vi "BotSpeak.Com.vi"(1 "To Send":string, 2 "Bot Settings in":T1) -> (3 "error out":errorcluster, 4 "Sent":string, 5 "Reply":string, 6 "Bot Settings out":T1)   [LabVIEW 2012]
uses:
  <userlib>/botspeak/VIs/Direct/BotSpeak_Control.ctl
  <userlib>/botspeak/VIs/SubVIs/BotSpeak_Globals.vi
panel:
  out "Numeric":i32
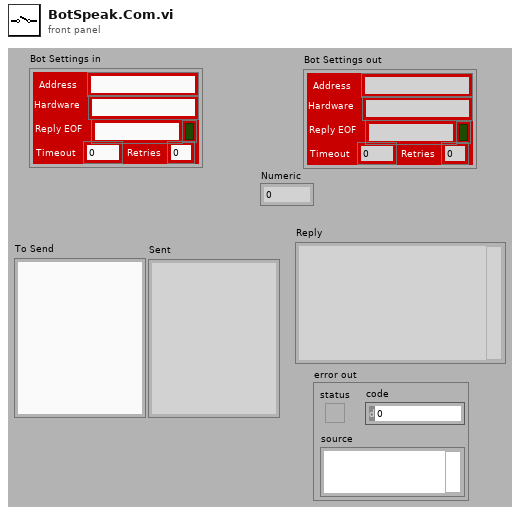
[diagram p1: front panel]
types:
  T1 = typedef "BotSpeak_Control.ctl" = cluster{"Address":string, "Reply EOF":string, "Hardware":string, "Retries":i8, "Timeout":i32, "Open?":bool}
  T2 = typedef "BotSpeak.HardwareSpecs.ctl" = cluster{"Hardware Name":string, "Hardware URL":string, "ComType":enum16{"Undefined", "HTTP", "Serial", "TCPIP", "Console"}, "TCP Port":i32, "DefaultAddress":string, "Retries":i32, "Translate":enum16{"None", "Tiny", "URAPI"}, "MaxScriptSize":i32, "MaxVarNumber":i32, "StartupWait":i32, "Patience":i32, "Startup Patience":i32, "Hardware Help":string, "Com Protocol":string, "Translator":cluster{"BotSpeak CMD":string, "CMD out":string}[], "Init Code":string, "Variable Format":enum16{"INT", "FLOAT", "FIXED"}, "username":string, "password":string}
  T3 = cluster{"BotSpeak CMD":string, "CMD out":string}[]
  T4 = enum16{"Undefined", "HTTP", "Serial", "TCPIP", "Console"}
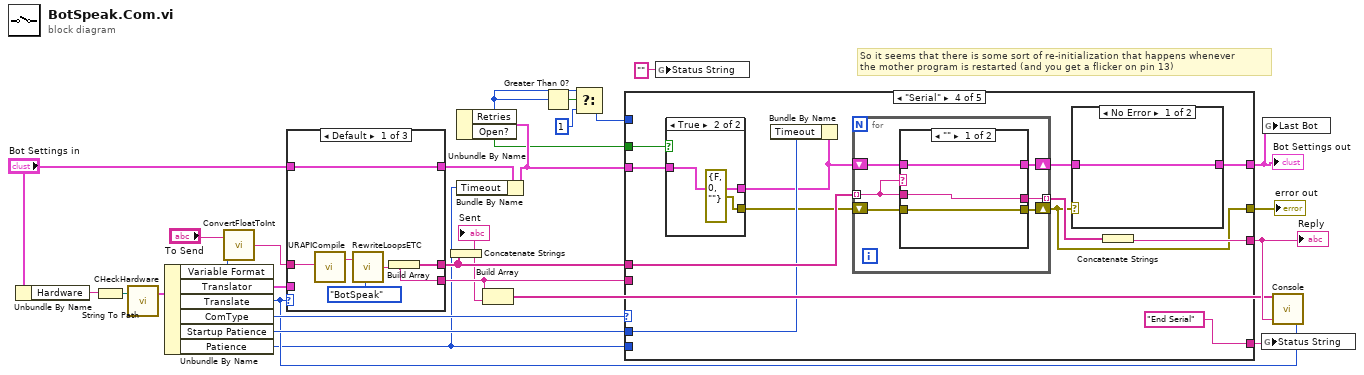
[diagram p0: block diagram]
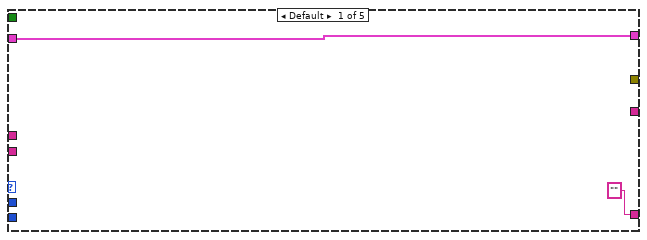
[diagram p2: hidden frame]
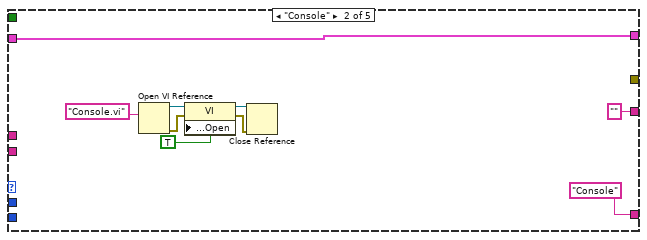
[diagram p3: hidden frame]
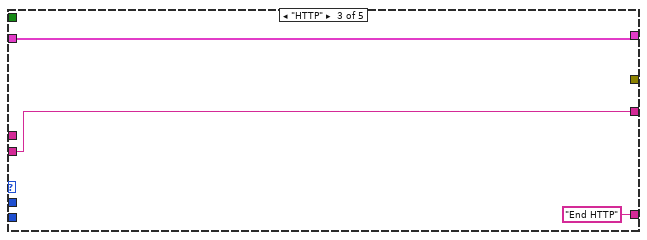
[diagram p4: hidden frame]
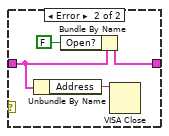
[diagram p5: hidden frame]
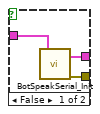
[diagram p6: hidden frame]
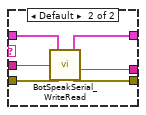
[diagram p7: hidden frame]
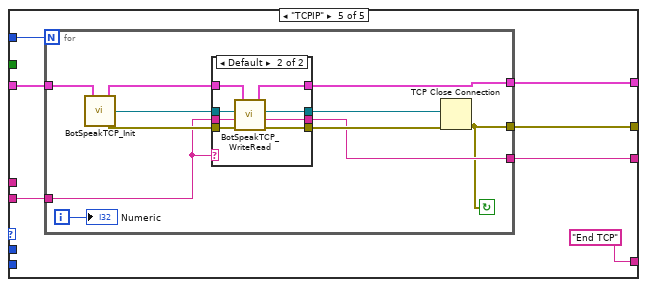
[diagram p8: hidden frame]
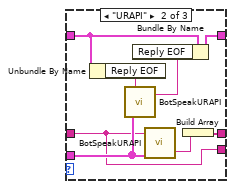
[diagram p10: hidden frame]
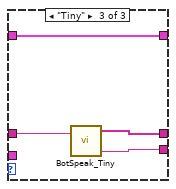
[diagram p11: hidden frame]
diagram:
  # "So it seems that there is some sort of re-initialization that happens whenever\nthe mother program is restarted (and you get a flicker on pin 13)"
  n1 = Unbundle By Name("Bot Settings in") -> ("Hardware"=w27:string)
  n2 = String To Path(string=w27) -> (path=w10:path)
  n3 = call <userlib>:"CHeckHardware.vi"("Hardware"=w10) -> ("HardwareSpecs"=w23:T2)  [unwired: 2 in]
  n4 = Unbundle By Name(w23) -> ("Variable Format"=w11:enum16{"INT", "FLOAT", "FIXED"}, "Translator"=w22:T3, "Translate"=w14:enum16{"None", "Tiny", "URAPI"}, "ComType"=w26:T4, "Startup Patience"=w21:i32, "Patience"=w8:i32)
  n5 = call <userlib>:"ConvertFloatToInt.vi"("Variable Format"=w11, "To Send in"="To Send") -> ("To Send out"=w12:string)
  n6 = case shown="Default" w14 {
    tunnel: w12 -> [w30 w35 w46]
    tunnel: [w33 w36 w45] -> w28
    tunnel: w22 -> [_ w41 _]
    tunnel: [w34 w39 w44] -> w9
    tunnel: "Bot Settings in" -> [w34 w40 w44]
    tunnel: [w31 w35 w43] -> w18
    frame Default {
      n7 = call <userlib>:"URAPICompile.vi"("Script"=w30) -> ("trimmed script"=w32:string)  [unwired: 1 in]
      n8 = call <userlib>:"RewriteLoopsETC.vi"("Type"=enum16{"Tiny", "BotSpeak"}."BotSpeak", "URAPI in"=w32) -> ("URAPI out"=w31:string)
      n9 = Build Array(w31) -> (w33:string[])
    }
    frame "URAPI" {
      n10 = Unbundle By Name(w40) -> ("Reply EOF"=w42:string)
      n11 = call <userlib>:"BotSpeakURAPI.vi"("Translator"=w41, "To Send"=w42) -> ("translated"=w38:string)  [unwired: 1 out]
      n12 = Bundle By Name(cluster=w40, "Reply EOF"=w38) -> (w39:T1)
      n13 = call <userlib>:"BotSpeakURAPI.vi"("Translator"=w41, "To Send"=w35) -> ("translated w \\n"=w37:string)  [unwired: 1 out]
      n14 = Build Array(w37) -> (w36:string[])
    }
    frame "Tiny" {
      n15 = call <userlib>:"BotSpeak_Tiny.vi"("URAPI"=w46) -> ("URAPI  2"=w43:string, "Tiny Lines"=w45:string[])  [unwired: 1 in, 1 out]
    }
  }
  n16 = Concatenate Strings(w28) -> (w17:string)
  "Sent" <- w17
  n17 = Bundle By Name(cluster=w9, "Timeout"=w8) -> (w6:T1)
  n18 = Unbundle By Name(w6) -> ("Retries"=w3:i8, "Open?"=w5:bool)
  n19 = Build Array(w18, w17) -> (w15:string[])
  n20 = Greater Than 0?(x=w3) -> (x > 0?=w4:bool)
  n21 = Select(t=w3, s=w4, f=i8 1) -> (s? t:f=w1:i8)
  n22 = case shown="\"Serial\"" w26 {
    tunnel: w28 -> [_ _ _ w72 _]
    tunnel: [_ "" ("data out") w59 w67 w100] -> w16
    tunnel: [_ _ _ w61 w102] -> w25
    tunnel: w6 -> [w48 w57 w60 w71 w103]
    tunnel: [w48 w57 w60 w64 w104] -> w7
    tunnel: w21 -> [_ _ _ w70 _]
    tunnel: ["" ("Status String") "Console" ("Status String") "End HTTP" ("Status String") "End Serial" ("Status String") "End TCP" ("Status String")] -> w20
    tunnel: w18 -> [_ _ w59 _ w99]
    tunnel: w8 -> [_ _ _ _ _]
    tunnel: w5 -> [_ _ _ w63 _]
    tunnel: w1 -> [_ _ _ _ w98]
    frame Default {
    }
    frame "Console" {
      n23 = Open VI Reference(vi path="Console.vi" ("Status String")) -> (vi reference=w54:refnum<vi>, error out=w53:errorcluster)  [unwired: 5 in]
      n24 = property class="VI"(reference=w54, error in=w53, "Front Panel.Open"=TRUE ("Front Panel Window:Open")) -> (reference out=w50:refnum<vi>, error out=w51:errorcluster)
      n25 = Close Reference(reference=w50, error in (no error)=w51) -> ()  [unwired: 1 out]
    }
    frame "HTTP" {
    }
    frame "Serial" {
      n26 = case shown="True" w63 {
        tunnel: w71 -> [w80 w82]
        tunnel: [w79 w82] -> w62
        tunnel: [w78 errorcluster {"status"=FALSE, "code"=0, "source"=""} ("error out")] -> w65
        frame False {
          n27 = call <userlib>:"BotSpeakSerial_Init.vi"("Bot Settings in"=w80) -> ("error out"=w78:errorcluster, "Bot Settings out"=w79:T1)  [unwired: 1 in]
        }
        frame True {
        }
      }
      n28 = Bundle By Name(cluster=w62, "Timeout"=w70) -> ()  [unwired: 1 out]
      n29 = for {
        tunnel: w72 -> [w83] mode=indexing
        tunnel: [w88] -> w68 mode=indexing
        shift-right: [w84] -> w66
        shift-left: w62 -> [w87]
        shift-right: [w85] -> w61
        shift-left: w65 -> [w86]
        n30 = case shown="\"\"" w83 {
          tunnel: w83 -> [w89 w97]
          tunnel: [w89 w96] -> w88
          tunnel: w87 -> [w91 w95]
          tunnel: w86 -> [w90 w94]
          tunnel: [w90 w93] -> w85
          tunnel: [w91 w92] -> w84
          frame "" {
          }
          frame Default {
            n31 = call <userlib>:"BotSpeakSerial_WriteRead.vi"("error In"=w94, "To Write"=w97, "Bot Settings in"=w95) -> ("error out"=w93:errorcluster, "Reply"=w96:string, "Bot Settings out"=w92:T1)  [unwired: 1 out]
          }
        }
      }
      n32 = case shown="No Error" w61 {
        tunnel: w66 -> [w73 w77]
        tunnel: [w73 w76] -> w64
        frame No Error {
        }
        frame Error {
          n33 = Unbundle By Name(w77) -> ("Address"=w75:string)
          n34 = Bundle By Name(cluster=w77, "Open?"=FALSE) -> (w76:T1)
          n35 = VISA Close(VISA resource name=w75) -> ()  [unwired: 1 in, 1 out]
        }
      }
      n36 = Concatenate Strings(w68) -> (w67:string)
    }
    frame "TCPIP" {
      n37 = for {
        N: w98 -> [_]
        tunnel: [w114] -> w104
        tunnel: w103 -> [w111]
        tunnel: [w106] -> w102
        tunnel: [w108] -> w100
        tunnel: w99 -> [w107]
        i -> [w105]
        stop <- w106 continue-if-true
        n38 = call <userlib>:"BotSpeakTCP_Init.vi"("Bot Settings in"=w111) -> ("error out"=w112:errorcluster, "connection ID"=w113:refnum<k5>, "Bot Settings out"=w115:T1)  [unwired: 1 in]
        n39 = case shown="Default" w107 {
          tunnel: w115 -> [w119 w127]
          tunnel: [w119 w126] -> w114
          tunnel: w113 -> [w118 w125]
          tunnel: w112 -> [w116 w124]
          tunnel: [w118 w123] -> w110
          tunnel: [w116 w122] -> w109
          tunnel: [w117 w121] -> w108
          tunnel: w107 -> [w117 w120]
          frame "" {
          }
          frame Default {
            n40 = call <userlib>:"BotSpeakTCP_WriteRead.vi"("error in"=w124, "To Send"=w120, "connection ID"=w125, "Bot Settings in"=w127) -> ("error out"=w122:errorcluster, "data out"=w121:string, "connection ID out"=w123:refnum<k5>, "Bot Settings out"=w126:T1)
          }
        }
        n41 = TCP Close Connection(connection ID=w110, error in (no error)=w109) -> (error out=w106:errorcluster)  [unwired: 1 in, 1 out]
        "Numeric" <- w105
      }
    }
  }
  "Reply" <- w16
  "error out" <- w25
  "Bot Settings out" <- w7
  n42 = global write "BotSpeak_Globals.vi" "Status String"("" ("Status String")) -> ()
  n43 = global write "BotSpeak_Globals.vi" "Status String"(w20) -> ()
  n44 = global write "BotSpeak_Globals.vi" "Last Bot"(w7) -> ()
  n45 = call <userlib>:"Console.vi"("Translate"=w14, "Reply"=w16, "Sent"=w15) -> ()  [unwired: 1 in, 2 out]
